vi "Operational Force Test.vi"(8 "error in (no error)":errorcluster, 10 "Model in":refnum<class "Model.lvclass">, 11 "Test Actuator State in":refnum<class "Test Actuator State.lvclass">) -> (0 "error out":errorcluster, 2 "Model out":refnum<class "Model.lvclass">, 3 "Test Actuator State out":refnum<class "Test Actuator State.lvclass">)   [LabVIEW 2016, in "Test Actuator State.lvclass"]
uses:
  Test Actuator State.lvclass
  Model/Model/Model.lvclass
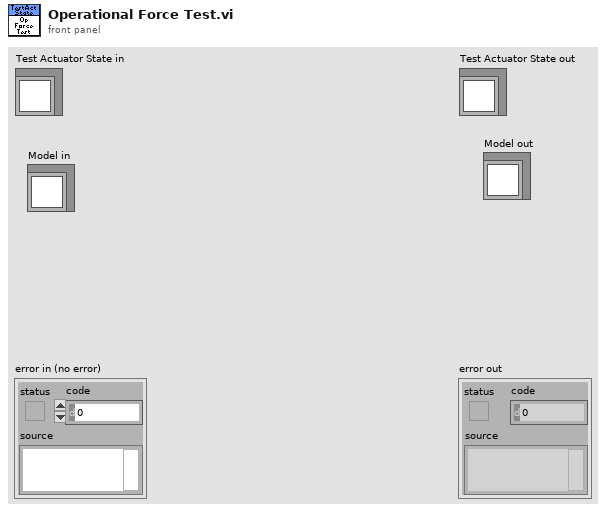
[diagram p1: front panel]
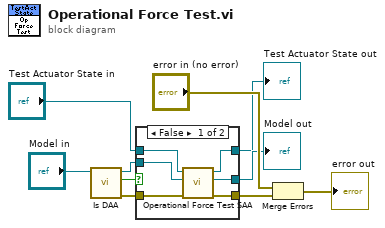
[diagram p0: block diagram]
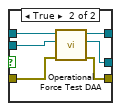
[diagram p2: hidden frame]
diagram:
  n1 = call "Is DAA.vi"("Model in"="Model in") -> ("error out"=w4:errorcluster, "IsDAA"=w7:bool, "Model out"=w6:refnum<class "Model.lvclass">)  [unwired: 8 in]
  n2 = case shown="False" w7 {
    tunnel: w6 -> [w14 w21]
    tunnel: "Test Actuator State in" -> [w16 w22]
    tunnel: w4 -> [w12 w20]
    tunnel: [w11 w19] -> w1
    tunnel: [w13 w18] -> w3
    tunnel: [w15 w17] -> w2
    frame False {
      n3 = call-dynamic "Operational Force Test SAA.vi"("error in (no error)"=w12, "Model in"=w14, "Test Actuator State in"=w16) -> ("error out"=w11:errorcluster, "Model out"=w13:refnum<class "Model.lvclass">, "Test Actuator State out"=w15:refnum<class "Test Actuator State.lvclass">)  [unwired: 6 in]
    }
    frame True {
      n4 = call-dynamic "Operational Force Test DAA.vi"("error in (no error)"=w20, "Model in"=w21, "Test Actuator State in"=w22) -> ("error out"=w19:errorcluster, "Model out"=w18:refnum<class "Model.lvclass">, "Test Actuator State out"=w17:refnum<class "Test Actuator State.lvclass">)  [unwired: 6 in]
    }
  }
  "Test Actuator State out" <- w2
  "Model out" <- w3
  n5 = Merge Errors("error in (no error)", w1) -> (→"error out":errorcluster)
